vi "Set Configuration.vi"(8 "error in (no error)":errorcluster, 11 "IO Class in":refnum<class "IO Class.lvclass">) -> (0 "error out":errorcluster, 3 "IO Class out":refnum<class "IO Class.lvclass">)   [LabVIEW 2015, in "IO Class.lvclass"]
uses:
  IO Class.lvclass
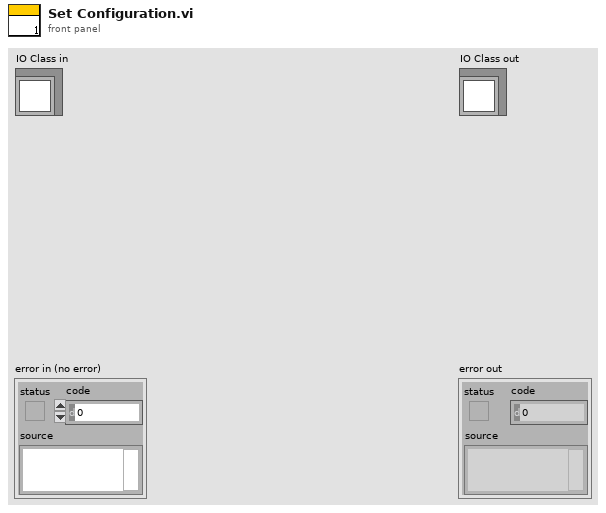
[diagram p1: front panel]
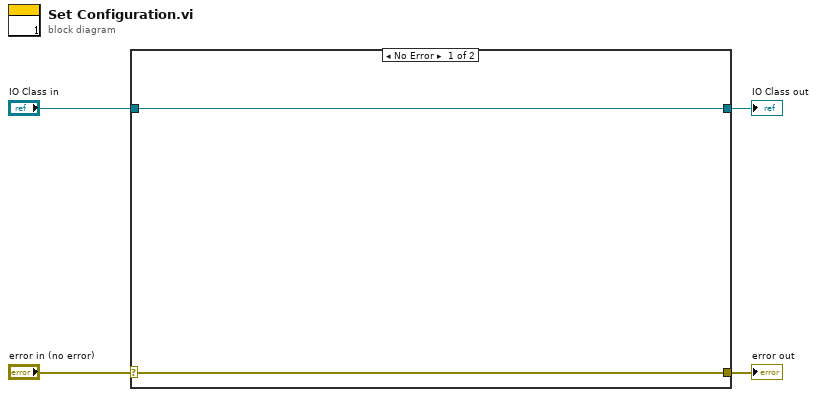
[diagram p0: block diagram]
diagram:
  n1 = case shown="No Error" "error in (no error)" {
    selector: "error in (no error)" -> [w5 w8]
    tunnel: [w5 w8] -> w3
    tunnel: [w6 w7] -> w1
    tunnel: "IO Class in" -> [w6 w7]
    frame No Error {
    }
    frame Error {
    }
  }
  "error out" <- w3
  "IO Class out" <- w1
